vi "Bin_Video_Viewer.vi"() -> ()   [LabVIEW 2013]
panel:
  out "Image":T1(plugin-control)
  out "Frame number":i32=4
  in  "stop":bool
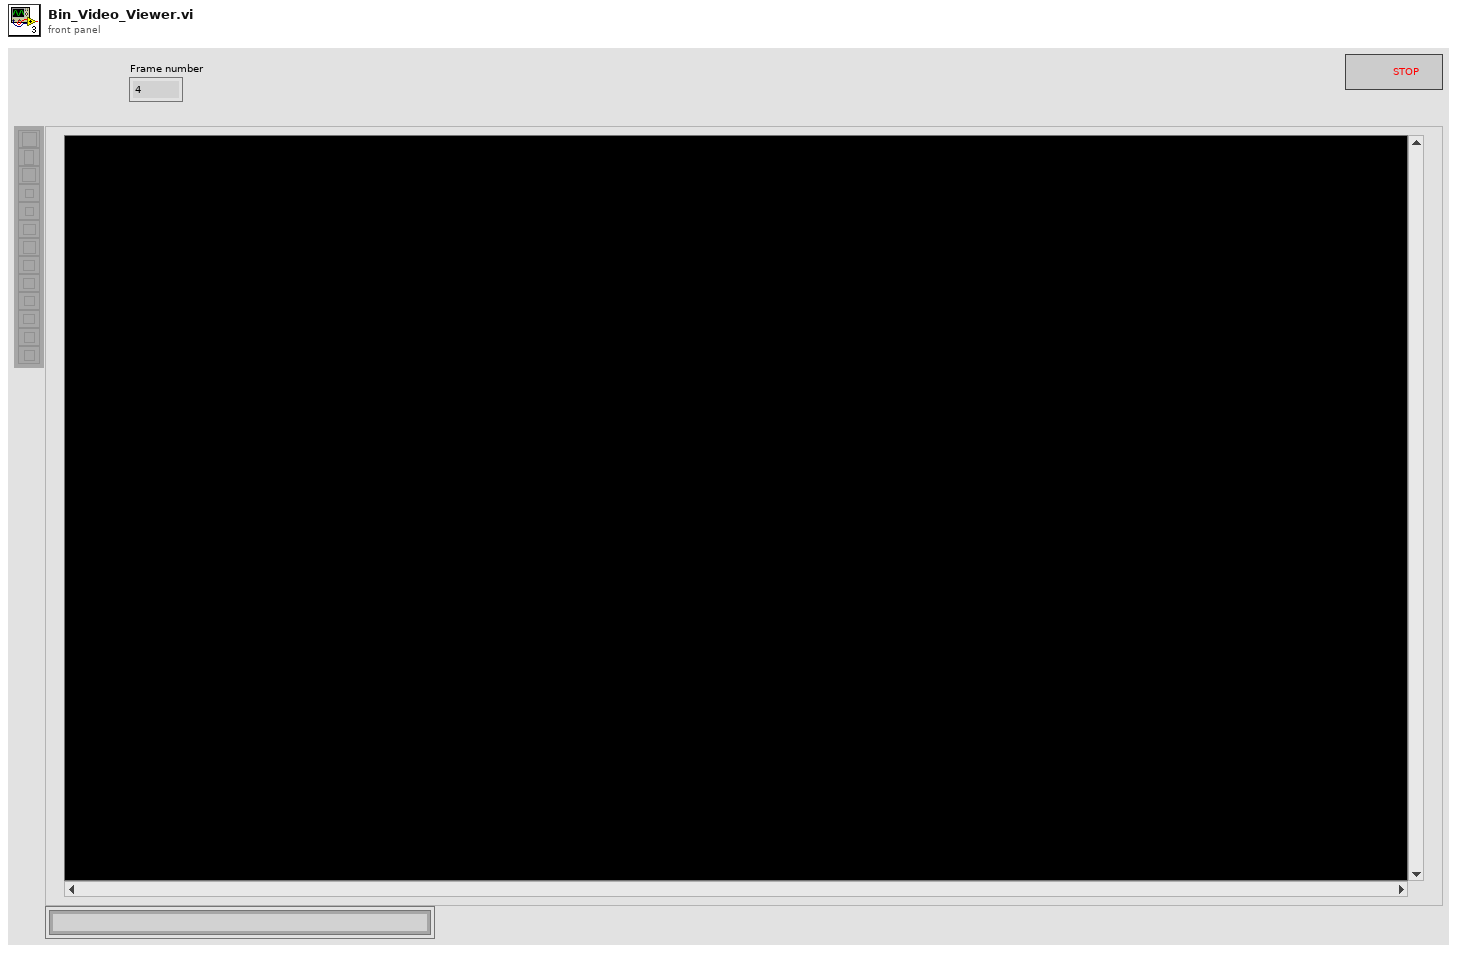
[diagram p1: front panel]
types:
  T1 = typedef "IMAQ Image.ctl" = refnum<image>
  T2 = typedef "Image Type" = u32
  T3 = enum16{"open", "replace", "create", "open or create", "replace or create", "replace or create with confirmation"}
  T4 = enum16{"big-endian, network order", "native, host order", "little-endian"}
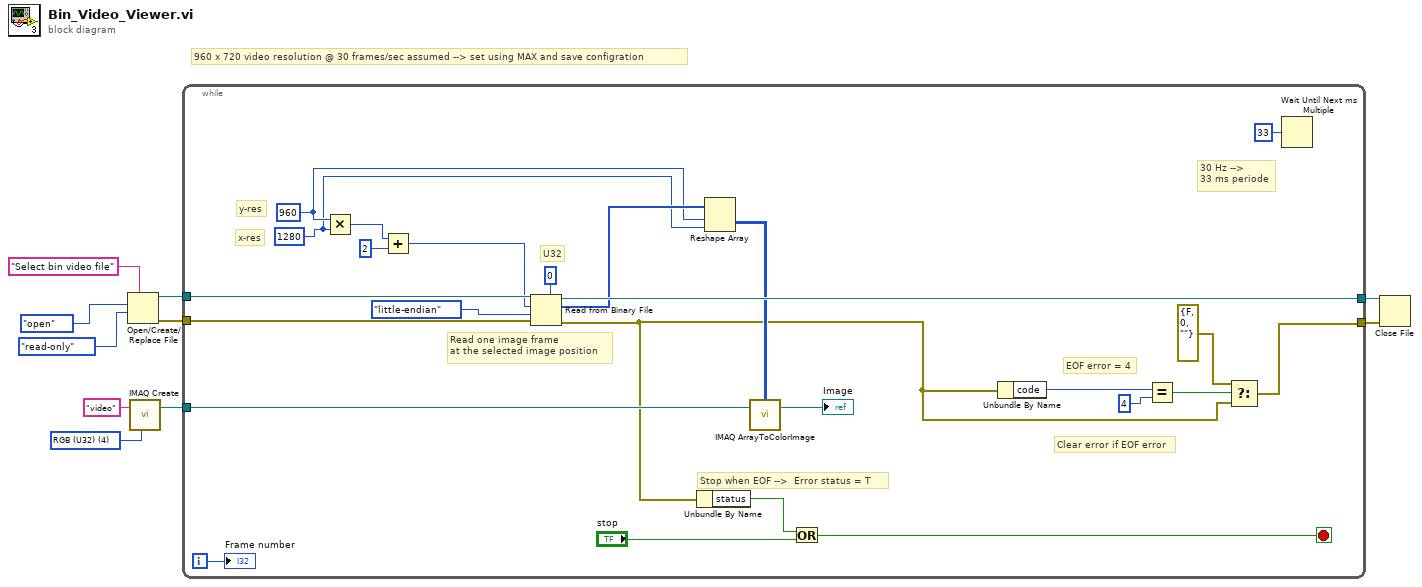
[diagram p0: block diagram]
diagram:
  w2 = T2 4 items=["Grayscale (U8)", "Grayscale (I16)", "Grayscale (SGL)", "Complex (CSG)", "RGB (U32)", "HSL (U32)", "RGB (U64)", "Grayscale (U16)"] ("Image Type")
  # "960 x 720 video resolution @ 30 frames/sec assumed --> set using MAX and save configration"
  n1 = Open/Create/Replace File(prompt="Select bin video file", operation (0:open)=T3."open", access (0:read/write)=enum16{"read/write", "read-only", "write-only"}."read-only") -> (refnum out=w8:refnum<file>, error out=w7:errorcluster)  [unwired: 3 in, 1 out]
  n2 = call "IMAQ Create"("Image Name"="video", "Image Type"=w2) -> ("New Image"=w1:T1)  [unwired: 3 in, 1 out]
  n3 = while {
    tunnel: w8 -> [w33]
    tunnel: w7 -> [w34]
    tunnel: [w31] -> w5
    tunnel: [w15] -> w4
    tunnel: w1 -> [w23]
    i -> [w22]
    stop <- w24 stop-if-true
    w28 = 1280
    w29 = 960
    # "Stop when EOF -->  Error status = T"
    # "30 Hz -->\n33 ms periode"
    # "Clear error if EOF error"
    # "EOF error = 4"
    # "y-res"
    # "x-res"
    # "Read one image frame \nat the selected image position"
    # "U32"
    n4 = Multiply(x=w29, y=w28) -> (x*y=w13:i32)
    n5 = Add(x=w13, y=2) -> (x+y=w12:i32)
    n6 = Read from Binary File(5:u32 0, 8:w34, 9:T4."little-endian" ("byte order (0:big-endian, network order)"), 10:w12, 11:w33) -> (0:w16:errorcluster, 2:w30:u32[], 3:w31:refnum<file>)  [unwired: 1 in, 1 out]
    n7 = Unbundle By Name(w16) -> ("status"=w26:bool)
    n8 = Reshape Array(w30, w29, w28) -> (w27:u32[][])
    n9 = call "IMAQ ArrayToColorImage"("Image Pixels (U32)"=w27, "Image"=w23) -> ("Image Out"=→"Image":T1)  [unwired: 3 in, 1 out]
    n10 = Or(x=w26, y="stop") -> (x .or. y?=w24:bool)
    n11 = Unbundle By Name(w16) -> ("code"=w20:i32)
    n12 = Equal?(x=w20, y=4) -> (x = y?=w18:bool)
    n13 = Select(t=errorcluster {"status"=FALSE, "code"=0, "source"=""}, s=w18, f=w16) -> (s? t:f=w15:errorcluster)
    n14 = Wait Until Next ms Multiple(millisecond multiple=u32 33) -> ()  [unwired: 1 out]
    "Frame number" <- w22
  }
  n15 = Close File(refnum=w5, error in=w4) -> ()  [unwired: 2 out]
